vi "LSMcontroller_v64_updatedwaveformhandling.vi"() -> ()   [LabVIEW 2015] (continued)
                        n3645 = local read "finite samples"() -> (w498:bool)
                        n3646 = local read "continuous"() -> (w501:bool)
                        n3647 = local read "wavdet"() -> (w502:bool)
                        n3648 = local read "# of frames"() -> (w500:i32)
                        n3649 = local read "maxbufferAI"() -> (w499:i32)
                        n3650 = local read "Override AI buffer"() -> (w495:bool)
                        n3651 = call "2pparameters.vi"("command"="get") -> ("params out"=w512:T10)  [unwired: 1 in]
                        n3652 = Bundle By Name(cluster=w512, "type"="X-Y-t movie", "avpp"=w515, "Angle Img"=w514, "Xpixels Img"=w510, "Vx-min Img"=w509, "VX-max Img"=w508, "Ypixels Img"=w506, "Vy-min Img"=w507, "Vy-max Img"=w503, "srate"=w497, "srate Img"=w497, "finite"=w498, "cont"=w501, "wavdet"=w502, "measpoints"=w500, "maxbufferAI"=w499, "Drawing Mode"=w513, "Vz-reset"=0.0, "AIoverride"=w495) -> (w504:T10)
                        n3653 = call "2pparameters.vi"("Params in"=w504, "command"="set") -> ()  [unwired: 1 out]
                      }
                      frame "X-Y-Z stack" {
                        n3654 = call "2pparameters.vi"("command"="get") -> ("params out"=w519:T10)  [unwired: 1 in]
                        n3655 = Bundle By Name(cluster=w519, "type"="X-Y-Z stack") -> (w517:T10)
                        n3656 = call "2pparameters.vi"("Params in"=w517, "command"="set") -> ()  [unwired: 1 out]
                      }
                      frame "Lifetime (scan)" {
                        n3657 = call "2pparameters.vi"("command"="get") -> ("params out"=w524:T10)  [unwired: 1 in]
                        n3658 = Bundle By Name(cluster=w524, "type"="Lifetime (scan)") -> (w522:T10)
                        n3659 = call "2pparameters.vi"("Params in"=w522, "command"="set") -> ()  [unwired: 1 out]
                      }
                      frame "Lifetime (contour)" {
                        n3660 = local read "Vy-min draw"() -> (w534:dbl)
                        n3661 = local read "Vy-max draw"() -> (w533:dbl)
                        n3662 = local read "Vx-min draw"() -> (w536:dbl)
                        n3663 = local read "Vx-max draw"() -> (w535:dbl)
                        n3664 = local read "xpixels ref"() -> (w532:i32)
                        n3665 = local read "ypixels ref"() -> (w531:i32)
                        n3666 = local read "ROI Type"() -> (w530:u16)
                        n3667 = local read "srateAODOtt"() -> (w541:dbl)
                        n3668 = local read "# of frames"() -> (w546:i32)
                        n3669 = local read "refreshtime"() -> (w538:dbl)
                        n3670 = local read "Pel"() -> (w529:dbl)
                        n3671 = local read "bin"() -> (w544:dbl)
                        n3672 = local read "Override AI buffer"() -> (w527:bool)
                        n3673 = local read "finite samples"() -> (w553:bool)
                        n3674 = local read "srateAODOtt"() -> (w540:dbl)
                        n3675 = local read "srateAODOtt"() -> (w547:dbl)
                        n3676 = local read "continuous"() -> (w552:bool)
                        n3677 = local read "Angle ref"() -> (w537:dbl)
                        n3678 = local read "wavdet"() -> (w554:bool)
                        n3679 = local read "Vx-ref"() -> (w549:dbl)
                        n3680 = local read "Vy-ref"() -> (w551:dbl)
                        n3681 = local read "avpp"() -> (w550:i32)
                        n3682 = call "tt_timeandsamples.vi"("bin"=w544, "refreshtime"=w538, "srateAODOtt"=w541, "tot#ofsamples"=w546) -> ("refreshrate"=w542:dbl, "refreshbuffer"=w543:i32, "timetracecycles"=w548:i32)  [unwired: 5 in]
                        n3683 = local read "bin"() -> (w545:dbl)
                        n3684 = call "2pparameters.vi"("command"="get") -> ("params out"=w557:T10)  [unwired: 1 in]
                        n3685 = Bundle By Name(cluster=w557, "Drawing Mode"=w530, "measpoints"=w546, "tt_cycles"=w548, "refreshbuffer"=w543, "refreshrate"=w542, "Vx-ref"=w549, "Vy-ref"=w551, "srate"=w540, "finite"=w553, "cont"=w552, "wavdet"=w554, "avpp"=w550, "srateAODO"=w547, "bufferAI"=w543, "bin"=w545, "Angle Img"=w537, "Vxminref"=w536, "Vxmaxref"=w535, "Vyminref"=w534, "Vymaxref"=w533, "Xpixels Img"=w532, "Ypixels Img"=w531, "Pel"=w529, "Vz-reset"=0.0, "AIoverride"=w527, "type"="Lifetime (contour)") -> (w555:T10)
                        n3686 = Reciprocal(x=w542) -> (1/x=w539:dbl)
                        n3687 = local write "refreshtime"(w539) -> ()
                        n3688 = call "2pparameters.vi"("Params in"=w555, "command"="set") -> ()  [unwired: 1 out]
                      }
                      frame "X-Y-Z-t movie" {
                      }
                      frame "linescan" {
                      }
                      frame "Timetrace" {
                        n3689 = local read "Vy-min draw"() -> (w567:dbl)
                        n3690 = local read "Vy-max draw"() -> (w566:dbl)
                        n3691 = local read "Vx-min draw"() -> (w569:dbl)
                        n3692 = local read "Vx-max draw"() -> (w568:dbl)
                        n3693 = local read "xpixels ref"() -> (w565:i32)
                        n3694 = local read "ypixels ref"() -> (w564:i32)
                        n3695 = local read "ROI Type"() -> (w563:u16)
                        n3696 = local read "srateAODOtt"() -> (w574:dbl)
                        n3697 = local read "# of frames"() -> (w579:i32)
                        n3698 = local read "refreshtime"() -> (w571:dbl)
                        n3699 = local read "Pel"() -> (w562:dbl)
                        n3700 = local read "bin"() -> (w577:dbl)
                        n3701 = local read "Override AI buffer"() -> (w560:bool)
                        n3702 = local read "finite samples"() -> (w586:bool)
                        n3703 = local read "srateAODOtt"() -> (w573:dbl)
                        n3704 = local read "srateAODOtt"() -> (w580:dbl)
                        n3705 = local read "continuous"() -> (w585:bool)
                        n3706 = local read "Angle ref"() -> (w570:dbl)
                        n3707 = local read "wavdet"() -> (w587:bool)
                        n3708 = local read "Vx-ref"() -> (w582:dbl)
                        n3709 = local read "Vy-ref"() -> (w584:dbl)
                        n3710 = local read "avpp"() -> (w583:i32)
                        n3711 = call "tt_timeandsamples.vi"("bin"=w577, "refreshtime"=w571, "srateAODOtt"=w574, "tot#ofsamples"=w579) -> ("refreshrate"=w575:dbl, "refreshbuffer"=w576:i32, "timetracecycles"=w581:i32)  [unwired: 5 in]
                        n3712 = local read "bin"() -> (w578:dbl)
                        n3713 = call "2pparameters.vi"("command"="get") -> ("params out"=w590:T10)  [unwired: 1 in]
                        n3714 = Bundle By Name(cluster=w590, "Drawing Mode"=w563, "measpoints"=w579, "tt_cycles"=w581, "refreshbuffer"=w576, "refreshrate"=w575, "Vx-ref"=w582, "Vy-ref"=w584, "srate"=w573, "finite"=w586, "cont"=w585, "wavdet"=w587, "avpp"=w583, "srateAODO"=w580, "bufferAI"=w576, "bin"=w578, "Angle Img"=w570, "Vxminref"=w569, "Vxmaxref"=w568, "Vyminref"=w567, "Vymaxref"=w566, "Xpixels Img"=w565, "Ypixels Img"=w564, "Pel"=w562, "Vz-reset"=0.0, "AIoverride"=w560, "type"="Timetrace") -> (w588:T10)
                        n3715 = Reciprocal(x=w575) -> (1/x=w572:dbl)
                        n3716 = local write "refreshtime"(w572) -> ()
                        n3717 = call "2pparameters.vi"("Params in"=w588, "command"="set") -> ()  [unwired: 1 out]
                      }
                      frame "Lifetime (point)" {
                      }
                    }
                  }
                  frame #1 {
                    w593 = FALSE ("wavdet")
                    n3718 = call "2pparameters.vi"("command"="get") -> ("params out"=w597:T10)  [unwired: 1 in]
                    n3719 = Bundle By Name(cluster=w597, "finite"=w593, "cont"=w593, "wavdet"=TRUE) -> (w594:T10)
                    n3720 = call "2pparameters.vi"("Params in"=w594, "command"="set") -> ()  [unwired: 1 out]
                  }
                  frame #2 {
                    n3721 = local read "DO channels"() -> (w604:u16)
                    n3722 = call "2pparameters.vi"("command"="get") -> ("params out"=w602:T10)  [unwired: 1 in]
                    n3723 = in-place {
                      in-place-border: w604 -> [w608]
                      in-place-border: [w605] -> w599
                      n3724 = in-place-cluster #51(w602) -> ("aDO"=w607:u32[])
                      n3725 = call "add channel to active arrayv2.vi"("line array in"=w607, "line to add"=w608) -> ("line array out"=w606:u32[], "addition"=w605:bool)  [unwired: 1 out]
                      n3726 = in-place-cluster #51("aDO"=w606) -> (w600:T10)
                    }
                    n3727 = local write "addDO"(w599) -> ()
                    n3728 = call "2pparameters.vi"("Params in"=w600, "command"="set") -> ()  [unwired: 1 out]
                  }
                  frame #3 {
                    n3729 = local read "addDO"() -> (w609:bool)
                    n3730 = case shown="True" w609 {
                      frame False {
                      }
                      frame True {
                        n3731 = call "Used AO lines.vi"() -> ("used AO names"=w613:string[], "used AO lines"=w615:tag[])  [unwired: 2 in]
                        n3732 = control-ref of="Analog Lines Plot"() -> (w614:refnum<vi>)
                        n3733 = control-ref of="Digital Lines Plot"() -> (w612:refnum<vi>)
                        n3734 = call "Used DO lines.vi"() -> ("used DO names"=w611:string[], "used DO lines"=w610:tag[])  [unwired: 2 in]
                        n3735 = local write "Analog Used Lines"(w615) -> ()
                        n3736 = local write "Analog Used Names"(w613) -> ()
                        n3737 = local write "Digital Used Lines"(w610) -> ()
                        n3738 = local write "Digital Used Names"(w611) -> ()
                        n3739 = call "prepDOWaveplot.vi"("DigitalGraph in"=w612, "used DO names"=w611) -> ()  [unwired: 1 in]
                        n3740 = call "prepAOWaveplot.vi"("WaveformGraph in"=w614, "Analog Used Names"=w613) -> ()  [unwired: 1 in]
                      }
                    }
                  }
                  frame #4 {
                    n3741 = local read "addDO"() -> (w616:bool)
                    n3742 = case shown="True" w616 {
                      frame False {
                      }
                      frame True {
                        n3743 = local read "Build digital waveform tabs"() -> (w617:enum32{"Simple", "Matlab"})
                        n3744 = case shown="\"Matlab\"" w617 {
                          frame "Simple", Default {
                            n3745 = local read "Meastab"() -> (w619:enum32{"X-Y Image", "Linescan", "Timetrace"})
                            n3746 = call "waveformparamsv2.vi"("command"="get") -> ("Params out"=w633:T14)  [unwired: 4 in, 2 out]
                            n3747 = case shown="\"Timetrace\"" w619 {
                              tunnel: [w635 w636] -> w618
                              frame "X-Y Image", Default {
                                n3748 = local read "Sampling rate"() -> (w635:dbl)
                              }
                              frame "Timetrace" {
                                n3749 = local read "srateAODOtt"() -> (w636:dbl)
                              }
                            }
                            n3750 = Unbundle By Name(w633) -> ("DO parameters"=w631:T17)
                            n3751 = local read "Digital padding value"() -> (w622:dbl)
                            n3752 = local read "Digital time offset (s)"() -> (w623:dbl)
                            n3753 = local read "Digital phase (s)"() -> (w625:dbl)
                            n3754 = local read "Digital Freq (Hz)"() -> (w624:dbl)
                            n3755 = local read "Digital DC (%)"() -> (w626:dbl)
                            n3756 = Index Array(array=w631, index=0) -> (element=w630:T18)
                            n3757 = Bundle By Name(cluster=w630, "Digital DC (%)"=w626, "Digital phase"=w625, "Digital Freq (Hz)"=w624, "Sampling frequency (Hz)"=w618, "Digital time offset (s)"=w623, "padding value"=w622, "matlab wave file"=path "", "DOtab"=0.0) -> (w628:T18)
                            n3758 = Build Array(w628) -> (w627:T17)
                            n3759 = call "waveformparamsv2.vi"("command"="add DO", "add DO"=w627) -> ()  [unwired: 3 in, 3 out]
                          }
                          frame "Matlab" {
                            w640 = 0.0 ("DOtab")
                            n3760 = local read "Meastab"() -> (w638:enum32{"X-Y Image", "Linescan", "Timetrace"})
                            n3761 = call "waveformparamsv2.vi"("command"="get") -> ("Params out"=w649:T14)  [unwired: 4 in, 2 out]
                            n3762 = case shown="\"Timetrace\"" w638 {
                              tunnel: [w651 w652] -> w637
                              frame "X-Y Image", Default {
                                n3763 = local read "Sampling rate"() -> (w651:dbl)
                              }
                              frame "Timetrace" {
                                n3764 = local read "srateAODOtt"() -> (w652:dbl)
                              }
                            }
                            n3765 = Unbundle By Name(w649) -> ("DO parameters"=w647:T17)
                            n3766 = local read "Matlab waveform path DO"() -> (w639:path)
                            n3767 = local read "Matlab padding value DO"() -> (w642:dbl)
                            n3768 = Index Array(array=w647, index=0) -> (element=w646:T18)
                            n3769 = Bundle By Name(cluster=w646, "Digital DC (%)"=w640, "Digital phase"=w640, "Digital Freq (Hz)"=w640, "Sampling frequency (Hz)"=w637, "Digital time offset (s)"=w640, "padding value"=w642, "matlab wave file"=w639, "DOtab"=1.0) -> (w644:T18)
                            n3770 = Build Array(w644) -> (w643:T17)
                            n3771 = call "waveformparamsv2.vi"("command"="add DO", "add DO"=w643) -> ()  [unwired: 3 in, 3 out]
                          }
                        }
                      }
                    }
                  }
                  frame #5 {
                    n3772 = local read "addDO"() -> (w654:bool)
                    n3773 = case shown="True" w654 {
                      tunnel: [_ w655] -> w653
                      frame False {
                      }
                      frame True {
                        n3774 = property on="refwf" class="Ring (strict)"() -> ("RingText.Text"=w660:string)  [unwired: 2 in, 2 out]
                        n3775 = call "waveformsDObuffer.vi"("command"="get") -> ("DO wf out"=w659:digitalwaveform[])  [unwired: 1 in]
                        n3776 = call "waveformsAObuffer.vi"("command"="get") -> ("AO wf out"=w657:waveform(dbl)[])  [unwired: 1 in]
                        n3777 = call "referfencesize.vi"("Digital waveforms in"=w659, "Analog waveforms in"=w657, "reference waveforms to"=w660) -> ("number of samples"=w655:i32)  [unwired: 2 in]
                      }
                    }
                  }
                  frame #6 {
                    n3778 = local read "Build digital waveform tabs"() -> (w671:enum32{"Simple", "Matlab"})
                    n3779 = call "waveformparamsv2.vi"("command"="get last DO") -> ("last DO"=w670:T18)  [unwired: 4 in, 2 out]
                    n3780 = local read "Meastab"() -> (w664:enum32{"X-Y Image", "Linescan", "Timetrace"})
                    n3781 = call "waveformsDObuffer.vi"("command"="get") -> ("DO wf out"=w669:digitalwaveform[])  [unwired: 1 in]
                    n3782 = case shown="\"Simple\", Default" w671 {
                      tunnel: w670 -> [w688 w690]
                      tunnel: w668 -> [w687 _]
                      tunnel: [w686 w689] -> w667
                      frame "Simple", Default {
                        n3783 = call "simple digital from wf params.vi"("waveform params"=w688, "number of samples"=w687) -> ("digital waveform"=w686:digitalwaveform)
                      }
                      frame "Matlab" {
                        n3784 = call "matlabDOwffromparam.vi"("waveform params"=w690) -> ("digital waveform"=w689:digitalwaveform)
                      }
                    }
                    n3785 = property on="refwf" class="Ring (strict)"() -> ("RingText.Text"=w674:string)  [unwired: 2 in, 2 out]
                    n3786 = case shown="\"Timetrace\"" w664 {
                      tunnel: [w683 w684] -> w663
                      frame "X-Y Image", Default {
                        n3787 = local read "Sampling rate"() -> (w683:dbl)
                      }
                      frame "Timetrace" {
                        n3788 = local read "srateAODOtt"() -> (w684:dbl)
                      }
                    }
                    n3789 = call "waveformsAObuffer.vi"("command"="get") -> ("AO wf out"=w682:waveform(dbl)[])  [unwired: 1 in]
                    n3790 = Build Array (concatenate)(w669, w667) -> (w673:digitalwaveform[])
                    n3791 = call "correctwaveformsizetemp.vi"("new sampling frequency (Hz)"=w663, "start"=FALSE, "reference waveforms to"=w674, "Analog waveforms in"=w682, "stop"=FALSE, "Digital waveforms in"=w673) -> ("analog wf out"=w677:waveform(dbl)[], "Digital wf out"=w675:digitalwaveform[], "measpoints"=w665:i32)
                    n3792 = local write "Analog Lines Plot"(w677) -> ()
                    n3793 = call "GetNumCamFramesv2.vi"("Digital Waveform Graph"=w675) -> ("Numeric"=w676:i32)  [unwired: 10 in]
                    n3794 = local write "Digital Lines Plot"(w675) -> ()
                    n3795 = call "waveformsAObuffer.vi"("AO wf in"=w677, "command"="set") -> ()  [unwired: 1 out]
                    n3796 = call "waveformsDObuffer.vi"("DO wf in"=w675, "command"="set") -> ()  [unwired: 1 out]
                    n3797 = local write "Total Camera Frames"(w676) -> ()
                    n3798 = local read "wavdet"() -> (w666:bool)
                    n3799 = case shown="True" w666 {
                      tunnel: w665 -> [_ w685]
                      frame False {
                      }
                      frame True {
                        n3800 = local write "# of frames"(w685) -> ()
                      }
                    }
                  }
                  frame #7 {
                    w692 = FALSE ("addAO")
                    n3801 = local read "Build digital waveform tabs"() -> (w691:enum32{"Simple", "Matlab"})
                    n3802 = case shown="\"Simple\", Default" w691 {
                      frame "Simple", Default {
                        n3803 = local write "not loadedDO"(FALSE ("not loadedDO")) -> ()
                      }
                      frame "Matlab" {
                        n3804 = local write "not loadedDOml"(FALSE ("not loadedDO")) -> ()
                      }
                    }
                    n3805 = local read "finite samples"() -> (w693:bool)
                    n3806 = local read "continuous"() -> (w694:bool)
                    n3807 = local read "wavdet"() -> (w695:bool)
                    n3808 = call "2pparameters.vi"("command"="get") -> ("params out"=w698:T10)  [unwired: 1 in]
                    n3809 = Bundle By Name(cluster=w698, "finite"=w693, "cont"=w694, "wavdet"=w695) -> (w696:T10)
                    n3810 = call "2pparameters.vi"("Params in"=w696, "command"="set") -> ()  [unwired: 1 out]
                    n3811 = local write "addDO"(w692) -> ()
                    n3812 = property on="Add DO wave" class="Bool (strict)"("Val(Sgnl)"=w692) -> ()  [unwired: 2 in, 2 out]
                  }
                }
              }
            }
          }
          event "DO channels": Value Change {
            n3813 = event-data() -> ()  [unwired: 1 in, 6 out]
            n3814 = local read "DO channels"() -> (w704:u16)
            n3815 = call "2pparameters.vi"("command"="get") -> ("params out"=w706:T10)  [unwired: 1 in]
            n3816 = Unbundle By Name(w706) -> ("aDO"=w705:u32[])
            n3817 = Search 1D Array(1D array=w705, element=w704) -> (index of element=w703:i32)  [unwired: 1 in]
            n3818 = Equal?(x=w703, y=-1.0) -> (x = y?=w702:bool)
            n3819 = case shown="False" w702 {
              tunnel: w703 -> [w721 _]
              frame False {
                n3820 = call "waveformparamsv2.vi"("command"="get") -> ("Params out"=w716:T14)  [unwired: 4 in, 2 out]
                n3821 = Unbundle By Name(w716) -> ("DO parameters"=w714:T17)
                n3822 = Index Array(array=w714, index=w721) -> (element=w720:T18)
                n3823 = Unbundle By Name(w720) -> ("Digital DC (%)"=w719:dbl, "Digital phase"=w718:dbl, "Digital Freq (Hz)"=w717:dbl, "Sampling frequency (Hz)"=w709:dbl, "Digital time offset (s)"=w713:dbl, "padding value"=w712:dbl, "matlab wave file"=w711:path, "DOtab"=w710:dbl)
                n3824 = local write "Build digital waveform tabs"(w710) -> ()
                n3825 = local write "Digital DC (%)"(w719) -> ()
                n3826 = local write "Matlab waveform path DO"(w711) -> ()
                n3827 = local write "Digital time offset (s)"(w713) -> ()
                n3828 = local write "Matlab padding value DO"(w712) -> ()
                n3829 = local write "Digital padding value"(w712) -> ()
                n3830 = local write "Sampling rate \ncurrent wf"(w709) -> ()
                n3831 = local write "Digital Freq (Hz)"(w717) -> ()
                n3832 = local write "Digital phase (s)"(w718) -> ()
              }
              frame True {
              }
            }
          }
          event "Rem DO wave": Value Change {
            n3833 = event-data() -> ("NewVal"=w722:bool)  [unwired: 1 in, 5 out]
            n3834 = case shown="True" w722 {
              frame False {
              }
              frame True {
                n3835 = stacked-sequence {
                  seq-local: [_ _ w828 _ _ _ _] -> [_ _ _ _ w847 w858 _]
                  frame #0 {
                    n3836 = local read "Measurement"() -> (w723:T4)
                    n3837 = case shown="\"linescan\"" w723 {
                      frame "X-Y-t movie", Default {
                        n3838 = local read "avpp"() -> (w744:i32)
                        n3839 = local read "Angle ref"() -> (w743:dbl)
                        n3840 = local read "ROI Type"() -> (w742:u16)
                        n3841 = local read "xpixels ref"() -> (w739:i32)
                        n3842 = local read "Vx-min ref"() -> (w738:dbl)
                        n3843 = local read "Vx-max ref"() -> (w737:dbl)
                        n3844 = local read "ypixels ref"() -> (w735:i32)
                        n3845 = local read "Vy-min ref"() -> (w736:dbl)
                        n3846 = local read "Vy-max ref"() -> (w732:dbl)
                        n3847 = local read "Sampling rate"() -> (w726:dbl)
                        n3848 = local read "finite samples"() -> (w727:bool)
                        n3849 = local read "continuous"() -> (w730:bool)
                        n3850 = local read "wavdet"() -> (w731:bool)
                        n3851 = local read "# of frames"() -> (w729:i32)
                        n3852 = local read "maxbufferAI"() -> (w728:i32)
                        n3853 = local read "Override AI buffer"() -> (w724:bool)
                        n3854 = call "2pparameters.vi"("command"="get") -> ("params out"=w741:T10)  [unwired: 1 in]
                        n3855 = Bundle By Name(cluster=w741, "type"="X-Y-t movie", "avpp"=w744, "Angle Img"=w743, "Xpixels Img"=w739, "Vx-min Img"=w738, "VX-max Img"=w737, "Ypixels Img"=w735, "Vy-min Img"=w736, "Vy-max Img"=w732, "srate"=w726, "srate Img"=w726, "finite"=w727, "cont"=w730, "wavdet"=w731, "measpoints"=w729, "maxbufferAI"=w728, "Drawing Mode"=w742, "Vz-reset"=0.0, "AIoverride"=w724) -> (w733:T10)
                        n3856 = call "2pparameters.vi"("Params in"=w733, "command"="set") -> ()  [unwired: 1 out]
                      }
                      frame "X-Y-Z stack" {
                        n3857 = call "2pparameters.vi"("command"="get") -> ("params out"=w748:T10)  [unwired: 1 in]
                        n3858 = Bundle By Name(cluster=w748, "type"="X-Y-Z stack") -> (w746:T10)
                        n3859 = call "2pparameters.vi"("Params in"=w746, "command"="set") -> ()  [unwired: 1 out]
                      }
                      frame "Lifetime (scan)" {
                        n3860 = call "2pparameters.vi"("command"="get") -> ("params out"=w753:T10)  [unwired: 1 in]
                        n3861 = Bundle By Name(cluster=w753, "type"="Lifetime (scan)") -> (w751:T10)
                        n3862 = call "2pparameters.vi"("Params in"=w751, "command"="set") -> ()  [unwired: 1 out]
                      }
                      frame "Lifetime (contour)" {
                        n3863 = local read "Vy-min draw"() -> (w763:dbl)
                        n3864 = local read "Vy-max draw"() -> (w762:dbl)
                        n3865 = local read "Vx-min draw"() -> (w765:dbl)
                        n3866 = local read "Vx-max draw"() -> (w764:dbl)
                        n3867 = local read "xpixels ref"() -> (w761:i32)
                        n3868 = local read "ypixels ref"() -> (w760:i32)
                        n3869 = local read "ROI Type"() -> (w759:u16)
                        n3870 = local read "srateAODOtt"() -> (w770:dbl)
                        n3871 = local read "# of frames"() -> (w775:i32)
                        n3872 = local read "refreshtime"() -> (w767:dbl)
                        n3873 = local read "Pel"() -> (w758:dbl)
                        n3874 = local read "bin"() -> (w773:dbl)
                        n3875 = local read "Override AI buffer"() -> (w756:bool)
                        n3876 = local read "finite samples"() -> (w782:bool)
                        n3877 = local read "srateAODOtt"() -> (w769:dbl)
                        n3878 = local read "srateAODOtt"() -> (w776:dbl)
                        n3879 = local read "continuous"() -> (w781:bool)
                        n3880 = local read "Angle ref"() -> (w766:dbl)
                        n3881 = local read "wavdet"() -> (w783:bool)
                        n3882 = local read "Vx-ref"() -> (w778:dbl)
                        n3883 = local read "Vy-ref"() -> (w780:dbl)
                        n3884 = local read "avpp"() -> (w779:i32)
                        n3885 = call "tt_timeandsamples.vi"("bin"=w773, "refreshtime"=w767, "srateAODOtt"=w770, "tot#ofsamples"=w775) -> ("refreshrate"=w771:dbl, "refreshbuffer"=w772:i32, "timetracecycles"=w777:i32)  [unwired: 5 in]
                        n3886 = local read "bin"() -> (w774:dbl)
                        n3887 = call "2pparameters.vi"("command"="get") -> ("params out"=w786:T10)  [unwired: 1 in]
                        n3888 = Bundle By Name(cluster=w786, "Drawing Mode"=w759, "measpoints"=w775, "tt_cycles"=w777, "refreshbuffer"=w772, "refreshrate"=w771, "Vx-ref"=w778, "Vy-ref"=w780, "srate"=w769, "finite"=w782, "cont"=w781, "wavdet"=w783, "avpp"=w779, "srateAODO"=w776, "bufferAI"=w772, "bin"=w774, "Angle Img"=w766, "Vxminref"=w765, "Vxmaxref"=w764, "Vyminref"=w763, "Vymaxref"=w762, "Xpixels Img"=w761, "Ypixels Img"=w760, "Pel"=w758, "Vz-reset"=0.0, "AIoverride"=w756, "type"="Lifetime (contour)") -> (w784:T10)
                        n3889 = Reciprocal(x=w771) -> (1/x=w768:dbl)
                        n3890 = local write "refreshtime"(w768) -> ()
                        n3891 = call "2pparameters.vi"("Params in"=w784, "command"="set") -> ()  [unwired: 1 out]
                      }
                      frame "X-Y-Z-t movie" {
                      }
                      frame "linescan" {
                      }
                      frame "Timetrace" {
                        n3892 = local read "Vy-min draw"() -> (w796:dbl)
                        n3893 = local read "Vy-max draw"() -> (w795:dbl)
                        n3894 = local read "Vx-min draw"() -> (w798:dbl)
                        n3895 = local read "Vx-max draw"() -> (w797:dbl)
                        n3896 = local read "xpixels ref"() -> (w794:i32)
                        n3897 = local read "ypixels ref"() -> (w793:i32)
                        n3898 = local read "ROI Type"() -> (w792:u16)
                        n3899 = local read "srateAODOtt"() -> (w803:dbl)
                        n3900 = local read "# of frames"() -> (w808:i32)
                        n3901 = local read "refreshtime"() -> (w800:dbl)
                        n3902 = local read "Pel"() -> (w791:dbl)
                        n3903 = local read "bin"() -> (w806:dbl)
                        n3904 = local read "Override AI buffer"() -> (w789:bool)
                        n3905 = local read "finite samples"() -> (w815:bool)
                        n3906 = local read "srateAODOtt"() -> (w802:dbl)
                        n3907 = local read "srateAODOtt"() -> (w809:dbl)
                        n3908 = local read "continuous"() -> (w814:bool)
                        n3909 = local read "Angle ref"() -> (w799:dbl)
                        n3910 = local read "wavdet"() -> (w816:bool)
                        n3911 = local read "Vx-ref"() -> (w811:dbl)
                        n3912 = local read "Vy-ref"() -> (w813:dbl)
                        n3913 = local read "avpp"() -> (w812:i32)
                        n3914 = call "tt_timeandsamples.vi"("bin"=w806, "refreshtime"=w800, "srateAODOtt"=w803, "tot#ofsamples"=w808) -> ("refreshrate"=w804:dbl, "refreshbuffer"=w805:i32, "timetracecycles"=w810:i32)  [unwired: 5 in]
                        n3915 = local read "bin"() -> (w807:dbl)
                        n3916 = call "2pparameters.vi"("command"="get") -> ("params out"=w819:T10)  [unwired: 1 in]
                        n3917 = Bundle By Name(cluster=w819, "Drawing Mode"=w792, "measpoints"=w808, "tt_cycles"=w810, "refreshbuffer"=w805, "refreshrate"=w804, "Vx-ref"=w811, "Vy-ref"=w813, "srate"=w802, "finite"=w815, "cont"=w814, "wavdet"=w816, "avpp"=w812, "srateAODO"=w809, "bufferAI"=w805, "bin"=w807, "Angle Img"=w799, "Vxminref"=w798, "Vxmaxref"=w797, "Vyminref"=w796, "Vymaxref"=w795, "Xpixels Img"=w794, "Ypixels Img"=w793, "Pel"=w791, "Vz-reset"=0.0, "AIoverride"=w789, "type"="Timetrace") -> (w817:T10)
                        n3918 = Reciprocal(x=w804) -> (1/x=w801:dbl)
                        n3919 = local write "refreshtime"(w801) -> ()
                        n3920 = call "2pparameters.vi"("Params in"=w817, "command"="set") -> ()  [unwired: 1 out]
                      }
                      frame "Lifetime (point)" {
                      }
                    }
                  }
                  frame #1 {
                    w822 = FALSE ("wavdet")
                    n3921 = call "2pparameters.vi"("command"="get") -> ("params out"=w826:T10)  [unwired: 1 in]
                    n3922 = Bundle By Name(cluster=w826, "finite"=w822, "cont"=w822, "wavdet"=TRUE) -> (w823:T10)
                    n3923 = call "2pparameters.vi"("Params in"=w823, "command"="set") -> ()  [unwired: 1 out]
                  }
                  frame #2 {
                    n3924 = local read "DO channels"() -> (w834:u16)
                    n3925 = call "2pparameters.vi"("command"="get") -> ("params out"=w832:T10)  [unwired: 1 in]
                    n3926 = in-place {
                      in-place-border: w834 -> [w839]
                      in-place-border: [w836] -> w829
                      in-place-border: [w835] -> w828
                      n3927 = in-place-cluster #52(w832) -> ("aDO"=w838:u32[])
                      n3928 = call "remove channel from active arrayv2.vi"("line array in"=w838, "line to remove"=w839) -> ("line array out"=w837:u32[], "removal"=w836:bool, "index"=w835:i32)
                      n3929 = in-place-cluster #52("aDO"=w837) -> (w830:T10)
                    }
                    n3930 = local write "remDO"(w829) -> ()
                    n3931 = call "2pparameters.vi"("Params in"=w830, "command"="set") -> ()  [unwired: 1 out]
                  }
                  frame #3 {
                    n3932 = local read "remDO"() -> (w840:bool)
                    n3933 = case shown="True" w840 {
                      frame False {
                      }
                      frame True {
                        n3934 = call "Used AO lines.vi"() -> ("used AO names"=w844:string[], "used AO lines"=w846:tag[])  [unwired: 2 in]
                        n3935 = local write "Analog Used Lines"(w846) -> ()
                        n3936 = local write "Analog Used Names"(w844) -> ()
                        n3937 = call "Used DO lines.vi"() -> ("used DO names"=w842:string[], "used DO lines"=w841:tag[])  [unwired: 2 in]
                        n3938 = control-ref of="Analog Lines Plot"() -> (w845:refnum<vi>)
                        n3939 = control-ref of="Digital Lines Plot"() -> (w843:refnum<vi>)
                        n3940 = local write "Digital Used Lines"(w841) -> ()
                        n3941 = local write "Digital Used Names"(w842) -> ()
                        n3942 = call "prepAOWaveplot.vi"("WaveformGraph in"=w845, "Analog Used Names"=w844) -> ()  [unwired: 1 in]
                        n3943 = call "prepDOWaveplot.vi"("DigitalGraph in"=w843, "used DO names"=w842) -> ()  [unwired: 1 in]
                      }
                    }
                  }
                  frame #4 {
                    n3944 = local read "remDO"() -> (w848:bool)
                    n3945 = case shown="True" w848 {
                      tunnel: w847 -> [_ w849]
                      frame False {
                      }
                      frame True {
                        n3946 = call "waveformparamsv2.vi"("command"="rem DO", "index"=w849) -> ()  [unwired: 3 in, 3 out]
                      }
                    }
                  }
                  frame #5 {
                    n3947 = local read "Meastab"() -> (w854:enum32{"X-Y Image", "Linescan", "Timetrace"})
                    n3948 = property on="refwf" class="Ring (strict)"() -> ("RingText.Text"=w861:string)  [unwired: 2 in, 2 out]
                    n3949 = call "waveformsDObuffer.vi"("command"="get") -> ("DO wf out"=w860:digitalwaveform[])  [unwired: 1 in]
                    n3950 = case shown="\"Timetrace\"" w854 {
                      tunnel: [w870 w871] -> w853
                      frame "X-Y Image", Default {
                        n3951 = local read "Sampling rate"() -> (w870:dbl)
                      }
                      frame "Timetrace" {
                        n3952 = local read "srateAODOtt"() -> (w871:dbl)
                      }
                    }
                    n3953 = call "waveformsAObuffer.vi"("command"="get") -> ("AO wf out"=w869:waveform(dbl)[])  [unwired: 1 in]
                    n3954 = Delete From Array(array=w860, length=1, index=w858) -> (array with subset deleted=w857:digitalwaveform[])  [unwired: 1 out]
                    n3955 = call "correctwaveformsizetemp.vi"("new sampling frequency (Hz)"=w853, "start"=FALSE, "reference waveforms to"=w861, "Analog waveforms in"=w869, "stop"=FALSE, "Digital waveforms in"=w857) -> ("analog wf out"=w864:waveform(dbl)[], "Digital wf out"=w862:digitalwaveform[], "measpoints"=w855:i32)
                    n3956 = local read "wavdet"() -> (w856:bool)
                    n3957 = call "waveformsAObuffer.vi"("AO wf in"=w864, "command"="set") -> ()  [unwired: 1 out]
                    n3958 = call "waveformsDObuffer.vi"("DO wf in"=w862, "command"="set") -> ()  [unwired: 1 out]
                    n3959 = local write "Analog Lines Plot"(w864) -> ()
                    n3960 = local write "Digital Lines Plot"(w862) -> ()
                    n3961 = call "GetNumCamFramesv2.vi"("Digital Waveform Graph"=w862) -> ("Numeric"=w863:i32)  [unwired: 10 in]
                    n3962 = case shown="True" w856 {
                      tunnel: w855 -> [_ w872]
                      frame False {
                      }
                      frame True {
                        n3963 = local write "# of frames"(w872) -> ()
                      }
                    }
                    n3964 = local write "Total Camera Frames"(w863) -> ()
                  }
                  frame #6 {
                    w873 = FALSE ("addAO")
                    n3965 = local read "finite samples"() -> (w874:bool)
                    n3966 = local read "continuous"() -> (w875:bool)
                    n3967 = local read "wavdet"() -> (w876:bool)
                    n3968 = local write "remDO"(w873) -> ()
                    n3969 = call "2pparameters.vi"("command"="get") -> ("params out"=w879:T10)  [unwired: 1 in]
                    n3970 = Bundle By Name(cluster=w879, "finite"=w874, "cont"=w875, "wavdet"=w876) -> (w877:T10)
                    n3971 = property on="Rem DO wave" class="Bool (strict)"("Val(Sgnl)"=w873) -> ()  [unwired: 2 in, 2 out]
                    n3972 = call "2pparameters.vi"("Params in"=w877, "command"="set") -> ()  [unwired: 1 out]
                  }
                }
              }
            }
          }
          event "load changed DO wave": Value Change {
            n3973 = event-data() -> ("NewVal"=w881:bool)  [unwired: 1 in, 5 out]
            n3974 = case shown="True" w881 {
              frame False {
              }
              frame True {
                n3975 = stacked-sequence {
                  seq-local: [_ _ w989 _ _] -> [_ _ _ w1006 _]
                  seq-local: [_ _ w988 _ _] -> [_ _ _ w1005 _]
                  frame #0 {
                    n3976 = local read "Measurement"() -> (w883:T4)
                    n3977 = local write "changeDO"(TRUE ("addAO")) -> ()
                    n3978 = case shown="\"X-Y-t movie\", Default" w883 {
                      frame "X-Y-t movie", Default {
                        n3979 = local read "avpp"() -> (w904:i32)
                        n3980 = local read "Angle ref"() -> (w903:dbl)
                        n3981 = local read "ROI Type"() -> (w902:u16)
                        n3982 = local read "xpixels ref"() -> (w899:i32)
                        n3983 = local read "Vx-min ref"() -> (w898:dbl)
                        n3984 = local read "Vx-max ref"() -> (w897:dbl)
                        n3985 = local read "ypixels ref"() -> (w895:i32)
                        n3986 = local read "Vy-min ref"() -> (w896:dbl)
                        n3987 = local read "Vy-max ref"() -> (w892:dbl)
                        n3988 = local read "Sampling rate"() -> (w886:dbl)
                        n3989 = local read "finite samples"() -> (w887:bool)
                        n3990 = local read "continuous"() -> (w890:bool)
                        n3991 = local read "wavdet"() -> (w891:bool)
                        n3992 = local read "# of frames"() -> (w889:i32)
                        n3993 = local read "maxbufferAI"() -> (w888:i32)
                        n3994 = local read "Override AI buffer"() -> (w884:bool)
                        n3995 = call "2pparameters.vi"("command"="get") -> ("params out"=w901:T10)  [unwired: 1 in]
                        n3996 = Bundle By Name(cluster=w901, "type"="X-Y-t movie", "avpp"=w904, "Angle Img"=w903, "Xpixels Img"=w899, "Vx-min Img"=w898, "VX-max Img"=w897, "Ypixels Img"=w895, "Vy-min Img"=w896, "Vy-max Img"=w892, "srate"=w886, "srate Img"=w886, "finite"=w887, "cont"=w890, "wavdet"=w891, "measpoints"=w889, "maxbufferAI"=w888, "Drawing Mode"=w902, "Vz-reset"=0.0, "AIoverride"=w884) -> (w893:T10)
                        n3997 = call "2pparameters.vi"("Params in"=w893, "command"="set") -> ()  [unwired: 1 out]
                      }
                      frame "X-Y-Z stack" {
                        n3998 = call "2pparameters.vi"("command"="get") -> ("params out"=w908:T10)  [unwired: 1 in]
                        n3999 = Bundle By Name(cluster=w908, "type"="X-Y-Z stack") -> (w906:T10)
                        n4000 = call "2pparameters.vi"("Params in"=w906, "command"="set") -> ()  [unwired: 1 out]
                      }
                      frame "Lifetime (scan)" {
                        n4001 = call "2pparameters.vi"("command"="get") -> ("params out"=w913:T10)  [unwired: 1 in]
                        n4002 = Bundle By Name(cluster=w913, "type"="Lifetime (scan)") -> (w911:T10)
                        n4003 = call "2pparameters.vi"("Params in"=w911, "command"="set") -> ()  [unwired: 1 out]
                      }
                      frame "Lifetime (contour)" {
                        n4004 = local read "Vy-min draw"() -> (w923:dbl)
                        n4005 = local read "Vy-max draw"() -> (w922:dbl)
                        n4006 = local read "Vx-min draw"() -> (w925:dbl)
                        n4007 = local read "Vx-max draw"() -> (w924:dbl)
                        n4008 = local read "xpixels ref"() -> (w921:i32)
                        n4009 = local read "ypixels ref"() -> (w920:i32)
                        n4010 = local read "ROI Type"() -> (w919:u16)
                        n4011 = local read "srateAODOtt"() -> (w930:dbl)
                        n4012 = local read "# of frames"() -> (w935:i32)
                        n4013 = local read "refreshtime"() -> (w927:dbl)
                        n4014 = local read "Pel"() -> (w918:dbl)
                        n4015 = local read "bin"() -> (w933:dbl)
                        n4016 = local read "Override AI buffer"() -> (w916:bool)
                        n4017 = local read "finite samples"() -> (w942:bool)
                        n4018 = local read "srateAODOtt"() -> (w929:dbl)
                        n4019 = local read "srateAODOtt"() -> (w936:dbl)
                        n4020 = local read "continuous"() -> (w941:bool)
                        n4021 = local read "Angle ref"() -> (w926:dbl)
                        n4022 = local read "wavdet"() -> (w943:bool)
                        n4023 = local read "Vx-ref"() -> (w938:dbl)
                        n4024 = local read "Vy-ref"() -> (w940:dbl)
                        n4025 = local read "avpp"() -> (w939:i32)
                        n4026 = call "tt_timeandsamples.vi"("bin"=w933, "refreshtime"=w927, "srateAODOtt"=w930, "tot#ofsamples"=w935) -> ("refreshrate"=w931:dbl, "refreshbuffer"=w932:i32, "timetracecycles"=w937:i32)  [unwired: 5 in]
                        n4027 = local read "bin"() -> (w934:dbl)
                        n4028 = call "2pparameters.vi"("command"="get") -> ("params out"=w946:T10)  [unwired: 1 in]
                        n4029 = Bundle By Name(cluster=w946, "Drawing Mode"=w919, "measpoints"=w935, "tt_cycles"=w937, "refreshbuffer"=w932, "refreshrate"=w931, "Vx-ref"=w938, "Vy-ref"=w940, "srate"=w929, "finite"=w942, "cont"=w941, "wavdet"=w943, "avpp"=w939, "srateAODO"=w936, "bufferAI"=w932, "bin"=w934, "Angle Img"=w926, "Vxminref"=w925, "Vxmaxref"=w924, "Vyminref"=w923, "Vymaxref"=w922, "Xpixels Img"=w921, "Ypixels Img"=w920, "Pel"=w918, "Vz-reset"=0.0, "AIoverride"=w916, "type"="Lifetime (contour)") -> (w944:T10)
                        n4030 = Reciprocal(x=w931) -> (1/x=w928:dbl)
                        n4031 = local write "refreshtime"(w928) -> ()
                        n4032 = call "2pparameters.vi"("Params in"=w944, "command"="set") -> ()  [unwired: 1 out]
                      }
                      frame "X-Y-Z-t movie" {
                      }
                      frame "linescan" {
                      }
                      frame "Timetrace" {
                        n4033 = local read "Vy-min draw"() -> (w956:dbl)
                        n4034 = local read "Vy-max draw"() -> (w955:dbl)
                        n4035 = local read "Vx-min draw"() -> (w958:dbl)
                        n4036 = local read "Vx-max draw"() -> (w957:dbl)
                        n4037 = local read "xpixels ref"() -> (w954:i32)
                        n4038 = local read "ypixels ref"() -> (w953:i32)
                        n4039 = local read "ROI Type"() -> (w952:u16)
                        n4040 = local read "srateAODOtt"() -> (w963:dbl)
                        n4041 = local read "# of frames"() -> (w968:i32)
                        n4042 = local read "refreshtime"() -> (w960:dbl)
                        n4043 = local read "Pel"() -> (w951:dbl)
                        n4044 = local read "bin"() -> (w966:dbl)
                        n4045 = local read "Override AI buffer"() -> (w949:bool)
                        n4046 = local read "finite samples"() -> (w975:bool)
                        n4047 = local read "srateAODOtt"() -> (w962:dbl)
                        n4048 = local read "srateAODOtt"() -> (w969:dbl)
                        n4049 = local read "continuous"() -> (w974:bool)
                        n4050 = local read "Angle ref"() -> (w959:dbl)
                        n4051 = local read "wavdet"() -> (w976:bool)
                        n4052 = local read "Vx-ref"() -> (w971:dbl)
                        n4053 = local read "Vy-ref"() -> (w973:dbl)
                        n4054 = local read "avpp"() -> (w972:i32)
                        n4055 = call "tt_timeandsamples.vi"("bin"=w966, "refreshtime"=w960, "srateAODOtt"=w963, "tot#ofsamples"=w968) -> ("refreshrate"=w964:dbl, "refreshbuffer"=w965:i32, "timetracecycles"=w970:i32)  [unwired: 5 in]
                        n4056 = local read "bin"() -> (w967:dbl)
                        n4057 = call "2pparameters.vi"("command"="get") -> ("params out"=w979:T10)  [unwired: 1 in]
                        n4058 = Bundle By Name(cluster=w979, "Drawing Mode"=w952, "measpoints"=w968, "tt_cycles"=w970, "refreshbuffer"=w965, "refreshrate"=w964, "Vx-ref"=w971, "Vy-ref"=w973, "srate"=w962, "finite"=w975, "cont"=w974, "wavdet"=w976, "avpp"=w972, "srateAODO"=w969, "bufferAI"=w965, "bin"=w967, "Angle Img"=w959, "Vxminref"=w958, "Vxmaxref"=w957, "Vyminref"=w956, "Vymaxref"=w955, "Xpixels Img"=w954, "Ypixels Img"=w953, "Pel"=w951, "Vz-reset"=0.0, "AIoverride"=w949, "type"="Timetrace") -> (w977:T10)
                        n4059 = Reciprocal(x=w964) -> (1/x=w961:dbl)
                        n4060 = local write "refreshtime"(w961) -> ()
                        n4061 = call "2pparameters.vi"("Params in"=w977, "command"="set") -> ()  [unwired: 1 out]
                      }
                      frame "Lifetime (point)" {
                      }
                    }
                  }
                  frame #1 {
                    w982 = FALSE ("wavdet")
                    n4062 = call "2pparameters.vi"("command"="get") -> ("params out"=w986:T10)  [unwired: 1 in]
                    n4063 = Bundle By Name(cluster=w986, "finite"=w982, "cont"=w982, "wavdet"=TRUE) -> (w983:T10)
                    n4064 = call "2pparameters.vi"("Params in"=w983, "command"="set") -> ()  [unwired: 1 out]
                  }
                  frame #2 {
                    n4065 = local read "DO channels"() -> (w991:u16)
                    n4066 = call "2pparameters.vi"("command"="get") -> ("params out"=w993:T10)  [unwired: 1 in]
                    n4067 = Unbundle By Name(w993) -> ("aDO"=w992:u32[])
                    n4068 = Search 1D Array(1D array=w992, element=w991) -> (index of element=w989:i32)  [unwired: 1 in]
                    n4069 = Greater?(x=w989, y=-1) -> (0:w988:bool)
                    n4070 = case shown="True" w988 {
                      tunnel: w989 -> [_ w1002]
                      frame False {
                      }
                      frame True {
                        n4071 = local read "Meastab"() -> (w996:enum32{"X-Y Image", "Linescan", "Timetrace"})
                        n4072 = local read "Digital padding value"() -> (w997:dbl)
                        n4073 = local read "Digital time offset (s)"() -> (w998:dbl)
                        n4074 = case shown="\"Timetrace\"" w996 {
                          tunnel: [w1003 w1004] -> w995
                          frame "X-Y Image", Default {
                            n4075 = local read "Sampling rate"() -> (w1003:dbl)
                          }
                          frame "Timetrace" {
                            n4076 = local read "srateAODOtt"() -> (w1004:dbl)
                          }
                        }
                        n4077 = local read "Digital Freq (Hz)"() -> (w1000:dbl)
                        n4078 = local read "Digital phase (s)"() -> (w999:dbl)
                        n4079 = local read "Digital DC (%)"() -> (w1001:dbl)
                        n4080 = call "replace DO wf param.vi"("Digital Freq (Hz)"=w1000, "Digital DC (%)"=w1001, "Digital phase"=w999, "Sampling frequency (Hz)"=w995, "Digital time offset (s)"=w998, "index of DO wave"=w1002, "padding value"=w997) -> ()  [unwired: 4 in]
                      }
                    }
                  }
                  frame #3 {
                    n4081 = case shown="True" w1005 {
                      tunnel: w1006 -> [_ w1013]
                      frame False {
                      }
                      frame True {
                        n4082 = local read "Meastab"() -> (w1010:enum32{"X-Y Image", "Linescan", "Timetrace"})
                        n4083 = call "waveformparamsv2.vi"("command"="get") -> ("Params out"=w1029:T14)  [unwired: 4 in, 2 out]
                        n4084 = Unbundle By Name(w1029) -> ("DO parameters"=w1028:T17)
                        n4085 = property on="refwf" class="Ring (strict)"() -> ("RingText.Text"=w1035:string)  [unwired: 2 in, 2 out]
                        n4086 = case shown="\"Timetrace\"" w1010 {
                          tunnel: [w1036 w1037] -> w1009
                          frame "X-Y Image", Default {
                            n4087 = local read "Sampling rate"() -> (w1036:dbl)
                          }
                          frame "Timetrace" {
                            n4088 = local read "srateAODOtt"() -> (w1037:dbl)
                          }
                        }
                        n4089 = call "waveformsAObuffer.vi"("command"="get") -> ("AO wf out"=w1033:waveform(dbl)[])  [unwired: 1 in]
                        n4090 = call "waveformsDObuffer.vi"("command"="get") -> ("DO wf out"=w1031:digitalwaveform[])  [unwired: 1 in]
                        n4091 = call "referfencesize.vi"("Digital waveforms in"=w1031, "Analog waveforms in"=w1033, "reference waveforms to"=w1035) -> ("number of samples"=w1026:i32)  [unwired: 2 in]
                        n4092 = Index Array(array=w1028, index=w1013) -> (element=w1027:T18)
                        n4093 = call "waveformsDObuffer.vi"("command"="get") -> ("DO wf out"=w1023:digitalwaveform[])  [unwired: 1 in]
                        n4094 = call "simple digital from wf params.vi"("waveform params"=w1027, "number of samples"=w1026) -> ("digital waveform"=w1025:digitalwaveform)
                        n4095 = property on="refwf" class="Ring (strict)"() -> ("RingText.Text"=w1015:string)  [unwired: 2 in, 2 out]
                        n4096 = Replace Array Subset(array=w1023, new element=w1025, index=w1013) -> (w1014:digitalwaveform[])
                        n4097 = call "waveformsAObuffer.vi"("command"="get") -> ("AO wf out"=w1022:waveform(dbl)[])  [unwired: 1 in]
                        n4098 = local read "wavdet"() -> (w1012:bool)
                        n4099 = call "correctwaveformsizetemp.vi"("new sampling frequency (Hz)"=w1009, "start"=FALSE, "reference waveforms to"=w1015, "Analog waveforms in"=w1022, "stop"=FALSE, "Digital waveforms in"=w1014) -> ("analog wf out"=w1018:waveform(dbl)[], "Digital wf out"=w1016:digitalwaveform[], "measpoints"=w1011:i32)
                        n4100 = local write "Analog Lines Plot"(w1018) -> ()
                        n4101 = call "GetNumCamFramesv2.vi"("Digital Waveform Graph"=w1016) -> ("Numeric"=w1017:i32)  [unwired: 10 in]
                        n4102 = local write "Digital Lines Plot"(w1016) -> ()
                        n4103 = case shown="True" w1012 {
                          tunnel: w1011 -> [_ w1038]
                          frame False {
                          }
                          frame True {
                            n4104 = local write "# of frames"(w1038) -> ()
                          }
                        }
                        n4105 = call "waveformsAObuffer.vi"("AO wf in"=w1018, "command"="set") -> ()  [unwired: 1 out]
                        n4106 = call "waveformsDObuffer.vi"("DO wf in"=w1016, "command"="set") -> ()  [unwired: 1 out]
                        n4107 = local write "Total Camera Frames"(w1017) -> ()
                      }
                    }
                  }
                  frame #4 {
                    w1040 = FALSE ("addAO")
                    n4108 = local read "finite samples"() -> (w1041:bool)
                    n4109 = local read "continuous"() -> (w1042:bool)
                    n4110 = local read "wavdet"() -> (w1043:bool)
                    n4111 = local write "changeDO"(w1040) -> ()
                    n4112 = property on="load changed DO wave" class="Bool (strict)"("Val(Sgnl)"=w1040) -> ()  [unwired: 2 in, 2 out]
                    n4113 = call "2pparameters.vi"("command"="get") -> ("params out"=w1046:T10)  [unwired: 1 in]
                    n4114 = Bundle By Name(cluster=w1046, "finite"=w1041, "cont"=w1042, "wavdet"=w1043) -> (w1044:T10)
                    n4115 = local write "not loadedDO"(FALSE ("not loadedDO")) -> ()
                    n4116 = call "2pparameters.vi"("Params in"=w1044, "command"="set") -> ()  [unwired: 1 out]
                  }
                }
              }
            }
          }
          event "refwf": Value Change {
            n4117 = event-data() -> ()  [unwired: 1 in, 6 out]
            n4118 = stacked-sequence {
              frame #0 {
                n4119 = local read "Measurement"() -> (w1048:T4)
                n4120 = case shown="\"X-Y-t movie\", Default" w1048 {
                  frame "X-Y-t movie", Default {
                    n4121 = local read "avpp"() -> (w1069:i32)
                    n4122 = local read "Angle ref"() -> (w1068:dbl)
                    n4123 = local read "ROI Type"() -> (w1067:u16)
                    n4124 = local read "xpixels ref"() -> (w1064:i32)
                    n4125 = local read "Vx-min ref"() -> (w1063:dbl)
                    n4126 = local read "Vx-max ref"() -> (w1062:dbl)
                    n4127 = local read "ypixels ref"() -> (w1060:i32)
                    n4128 = local read "Vy-min ref"() -> (w1061:dbl)
                    n4129 = local read "Vy-max ref"() -> (w1057:dbl)
                    n4130 = local read "Sampling rate"() -> (w1051:dbl)
                    n4131 = local read "finite samples"() -> (w1052:bool)
                    n4132 = local read "continuous"() -> (w1055:bool)
                    n4133 = local read "wavdet"() -> (w1056:bool)
                    n4134 = local read "# of frames"() -> (w1054:i32)
                    n4135 = local read "maxbufferAI"() -> (w1053:i32)
                    n4136 = local read "Override AI buffer"() -> (w1049:bool)
                    n4137 = call "2pparameters.vi"("command"="get") -> ("params out"=w1066:T10)  [unwired: 1 in]
                    n4138 = Bundle By Name(cluster=w1066, "type"="X-Y-t movie", "avpp"=w1069, "Angle Img"=w1068, "Xpixels Img"=w1064, "Vx-min Img"=w1063, "VX-max Img"=w1062, "Ypixels Img"=w1060, "Vy-min Img"=w1061, "Vy-max Img"=w1057, "srate"=w1051, "srate Img"=w1051, "finite"=w1052, "cont"=w1055, "wavdet"=w1056, "measpoints"=w1054, "maxbufferAI"=w1053, "Drawing Mode"=w1067, "Vz-reset"=0.0, "AIoverride"=w1049) -> (w1058:T10)
                    n4139 = call "2pparameters.vi"("Params in"=w1058, "command"="set") -> ()  [unwired: 1 out]
                  }
                  frame "X-Y-Z stack" {
                    n4140 = call "2pparameters.vi"("command"="get") -> ("params out"=w1073:T10)  [unwired: 1 in]
                    n4141 = Bundle By Name(cluster=w1073, "type"="X-Y-Z stack") -> (w1071:T10)
                    n4142 = call "2pparameters.vi"("Params in"=w1071, "command"="set") -> ()  [unwired: 1 out]
                  }
                  frame "Lifetime (scan)" {
                    n4143 = call "2pparameters.vi"("command"="get") -> ("params out"=w1078:T10)  [unwired: 1 in]
                    n4144 = Bundle By Name(cluster=w1078, "type"="Lifetime (scan)") -> (w1076:T10)
                    n4145 = call "2pparameters.vi"("Params in"=w1076, "command"="set") -> ()  [unwired: 1 out]
                  }
                  frame "Lifetime (contour)" {
                    n4146 = local read "Vy-min draw"() -> (w1088:dbl)
                    n4147 = local read "Vy-max draw"() -> (w1087:dbl)
                    n4148 = local read "Vx-min draw"() -> (w1090:dbl)
                    n4149 = local read "Vx-max draw"() -> (w1089:dbl)
                    n4150 = local read "xpixels ref"() -> (w1086:i32)
                    n4151 = local read "ypixels ref"() -> (w1085:i32)
                    n4152 = local read "ROI Type"() -> (w1084:u16)
                    n4153 = local read "srateAODOtt"() -> (w1095:dbl)
                    n4154 = local read "# of frames"() -> (w1100:i32)
                    n4155 = local read "refreshtime"() -> (w1092:dbl)
                    n4156 = local read "Pel"() -> (w1083:dbl)
                    n4157 = local read "bin"() -> (w1098:dbl)
                    n4158 = local read "Override AI buffer"() -> (w1081:bool)
                    n4159 = local read "finite samples"() -> (w1107:bool)
                    n4160 = local read "srateAODOtt"() -> (w1094:dbl)
                    n4161 = local read "srateAODOtt"() -> (w1101:dbl)
                    n4162 = local read "continuous"() -> (w1106:bool)
                    n4163 = local read "Angle ref"() -> (w1091:dbl)
                    n4164 = local read "wavdet"() -> (w1108:bool)
                    n4165 = local read "Vx-ref"() -> (w1103:dbl)
                    n4166 = local read "Vy-ref"() -> (w1105:dbl)
                    n4167 = local read "avpp"() -> (w1104:i32)
                    n4168 = call "tt_timeandsamples.vi"("bin"=w1098, "refreshtime"=w1092, "srateAODOtt"=w1095, "tot#ofsamples"=w1100) -> ("refreshrate"=w1096:dbl, "refreshbuffer"=w1097:i32, "timetracecycles"=w1102:i32)  [unwired: 5 in]
                    n4169 = local read "bin"() -> (w1099:dbl)
                    n4170 = call "2pparameters.vi"("command"="get") -> ("params out"=w1111:T10)  [unwired: 1 in]
                    n4171 = Bundle By Name(cluster=w1111, "Drawing Mode"=w1084, "measpoints"=w1100, "tt_cycles"=w1102, "refreshbuffer"=w1097, "refreshrate"=w1096, "Vx-ref"=w1103, "Vy-ref"=w1105, "srate"=w1094, "finite"=w1107, "cont"=w1106, "wavdet"=w1108, "avpp"=w1104, "srateAODO"=w1101, "bufferAI"=w1097, "bin"=w1099, "Angle Img"=w1091, "Vxminref"=w1090, "Vxmaxref"=w1089, "Vyminref"=w1088, "Vymaxref"=w1087, "Xpixels Img"=w1086, "Ypixels Img"=w1085, "Pel"=w1083, "Vz-reset"=0.0, "AIoverride"=w1081, "type"="Lifetime (contour)") -> (w1109:T10)
                    n4172 = Reciprocal(x=w1096) -> (1/x=w1093:dbl)
                    n4173 = local write "refreshtime"(w1093) -> ()
                    n4174 = call "2pparameters.vi"("Params in"=w1109, "command"="set") -> ()  [unwired: 1 out]
                  }
                  frame "X-Y-Z-t movie" {
                  }
                  frame "linescan" {
                  }
                  frame "Timetrace" {
                    n4175 = local read "Vy-min draw"() -> (w1121:dbl)
                    n4176 = local read "Vy-max draw"() -> (w1120:dbl)
                    n4177 = local read "Vx-min draw"() -> (w1123:dbl)
                    n4178 = local read "Vx-max draw"() -> (w1122:dbl)
                    n4179 = local read "xpixels ref"() -> (w1119:i32)
                    n4180 = local read "ypixels ref"() -> (w1118:i32)
                    n4181 = local read "ROI Type"() -> (w1117:u16)
                    n4182 = local read "srateAODOtt"() -> (w1128:dbl)
                    n4183 = local read "# of frames"() -> (w1133:i32)
                    n4184 = local read "refreshtime"() -> (w1125:dbl)
                    n4185 = local read "Pel"() -> (w1116:dbl)
                    n4186 = local read "bin"() -> (w1131:dbl)
                    n4187 = local read "Override AI buffer"() -> (w1114:bool)
                    n4188 = local read "finite samples"() -> (w1140:bool)
                    n4189 = local read "srateAODOtt"() -> (w1127:dbl)
                    n4190 = local read "srateAODOtt"() -> (w1134:dbl)
                    n4191 = local read "continuous"() -> (w1139:bool)
                    n4192 = local read "Angle ref"() -> (w1124:dbl)
                    n4193 = local read "wavdet"() -> (w1141:bool)
                    n4194 = local read "Vx-ref"() -> (w1136:dbl)
                    n4195 = local read "Vy-ref"() -> (w1138:dbl)
                    n4196 = local read "avpp"() -> (w1137:i32)
                    n4197 = call "tt_timeandsamples.vi"("bin"=w1131, "refreshtime"=w1125, "srateAODOtt"=w1128, "tot#ofsamples"=w1133) -> ("refreshrate"=w1129:dbl, "refreshbuffer"=w1130:i32, "timetracecycles"=w1135:i32)  [unwired: 5 in]
                    n4198 = local read "bin"() -> (w1132:dbl)
                    n4199 = call "2pparameters.vi"("command"="get") -> ("params out"=w1144:T10)  [unwired: 1 in]
                    n4200 = Bundle By Name(cluster=w1144, "Drawing Mode"=w1117, "measpoints"=w1133, "tt_cycles"=w1135, "refreshbuffer"=w1130, "refreshrate"=w1129, "Vx-ref"=w1136, "Vy-ref"=w1138, "srate"=w1127, "finite"=w1140, "cont"=w1139, "wavdet"=w1141, "avpp"=w1137, "srateAODO"=w1134, "bufferAI"=w1130, "bin"=w1132, "Angle Img"=w1124, "Vxminref"=w1123, "Vxmaxref"=w1122, "Vyminref"=w1121, "Vymaxref"=w1120, "Xpixels Img"=w1119, "Ypixels Img"=w1118, "Pel"=w1116, "Vz-reset"=0.0, "AIoverride"=w1114, "type"="Timetrace") -> (w1142:T10)
                    n4201 = Reciprocal(x=w1129) -> (1/x=w1126:dbl)
                    n4202 = local write "refreshtime"(w1126) -> ()
                    n4203 = call "2pparameters.vi"("Params in"=w1142, "command"="set") -> ()  [unwired: 1 out]
                  }
                  frame "Lifetime (point)" {
                  }
                }
              }
              frame #1 {
                w1147 = FALSE ("wavdet")
                n4204 = call "2pparameters.vi"("command"="get") -> ("params out"=w1151:T10)  [unwired: 1 in]
                n4205 = Bundle By Name(cluster=w1151, "finite"=w1147, "cont"=w1147, "wavdet"=TRUE) -> (w1148:T10)
                n4206 = call "2pparameters.vi"("Params in"=w1148, "command"="set") -> ()  [unwired: 1 out]
              }
              frame #2 {
                n4207 = local read "Meastab"() -> (w1156:enum32{"X-Y Image", "Linescan", "Timetrace"})
                n4208 = property on="refwf" class="Ring (strict)"() -> ("RingText.Text"=w1159:string)  [unwired: 2 in, 2 out]
                n4209 = case shown="\"Timetrace\"" w1156 {
                  tunnel: [w1169 w1170] -> w1155
                  frame "X-Y Image", Default {
                    n4210 = local read "Sampling rate"() -> (w1169:dbl)
                  }
                  frame "Timetrace" {
                    n4211 = local read "srateAODOtt"() -> (w1170:dbl)
                  }
                }
